vi "MessageName.vi"() -> (2 "MessageName":string)   [LabVIEW 2020, in "TcpClientInfo.lvlib"]
uses:
  TcpClientInfo.lvlib
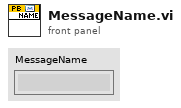
[diagram p1: front panel]
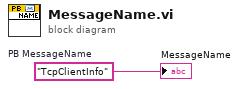
[diagram p0: block diagram]
diagram:
  w1 = "TcpClientInfo"  # PB MessageName
  "MessageName" <- w1
